vi "Write Section.vi"   [LabVIEW 2020, in "Generic Config Handling.lvlib"]
doc: "This vi writes the cluster as a section in the config file. \n\nIf section name is not wired then the default is to use the name of the cluster.\n\nEach element of the cluster becomes a key, therefore it must be named, and they should be unique and not include any special characters (spaces are allowed and are replaced by_)\n\nYou cannot nest clusters and only simple datatypes are allowed. 1D and 2D arrays are allowed. They are stored as a single element with columns delimited by semicolons and rows delimited by commas. 1D arrays are stored as a single row (ie. comma delimited). \n\nEnums are stored as U32s."
uses:
  Generic Config Handling.lvlib
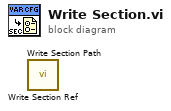
[diagram p0: block diagram]
diagram:
  n1 = call "Write Section Ref.vi"() -> ()  [unwired: 10 in, 2 out]
  n2 = call "Write Section Path.vi"() -> ()  [unwired: 9 in, 3 out]
